vi "Callback Change Channel.vi"(8 "error in (no error)":errorcluster, 9 "old values":string[][](array[string]), 10 "object ref in":T1, 11 "Cluster":T2) -> (0 "error out":errorcluster, 6 "Variant":variant)   [LabVIEW 2013, in "Modbus Module editor node.lvclass"]
uses:
  Modbus Module editor node.lvclass
  <vilib>/NI/DCAF Table API/Table Manager/Cell Change.ctl
  <vilib>/NI/DCAF Table API/Table Manager/object ref.ctl
  <vilib>/NI/DCAF/Tag Editor Core/Configuration Editor/Classes/Engine Parent/Engine Parent Editor Node.lvclass
  <vilib>/NI/DCAF/Tag Editor Core/Configuration Editor/Classes/Module editor node/module editor node.lvclass
  module/configuration/Modbus Module configuration.lvclass
  <vilib>/NI/Configuration Framework/serializable configuration/NISE_CEF_serializable configuration.lvclass/NISE_CEF_serializable configuration.ctl
  <vilib>/NI/Tag Bus/tag/tag descriptor.lvclass/tag descriptor.ctl
  <vilib>/Utility/LVClass/Get LV Class Name.vi
  <vilib>/NI/Configuration Framework/error generator/NISE_error generator.vi
  <vilib>/NI/Module Execution Interface/Engine Configuration/engine configuration.lvclass
  <vilib>/NI/Configuration Framework/serializable configuration/NISE_CEF_serializable configuration.lvclass
  <vilib>/NI/Tag Bus/tag/tag descriptor.lvclass
  <vilib>/NI/DCAF Table API/Table Manager.lvlib
  <vilib>/NI/DCAF Table API/Table Manager/Table Manager.lvclass
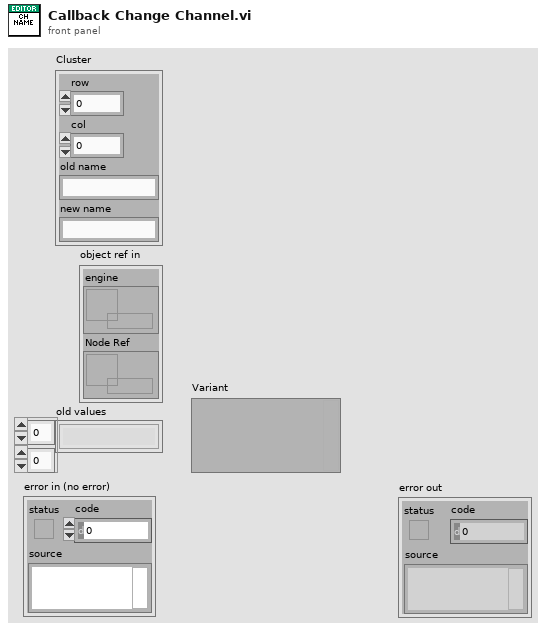
[diagram p1: front panel]
types:
  T1 = typedef "Table Manager.lvlib/Table Manager.lvclass/object ref.ctl" = cluster{"engine":refnum<data-value>, "Node Ref":refnum<data-value>}
  T2 = typedef "Table Manager.lvlib/Cell Change.ctl" = cluster{"row":i32, "col":i32, "old name":string, "new name":string}
  T3 = typedef "Modbus Module configuration.lvclass/Line.ctl" = refnum<class "Modbus Module Channel.lvclass">
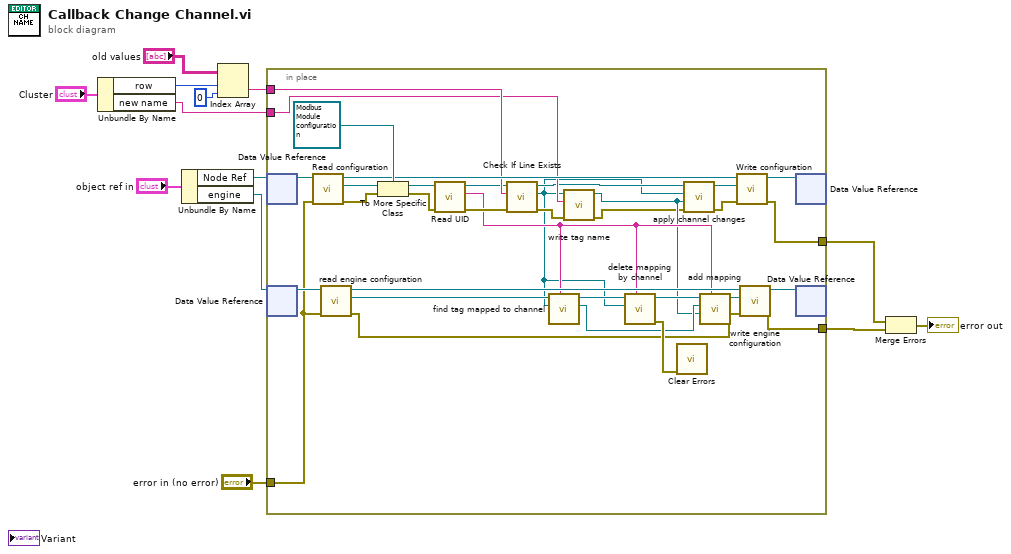
[diagram p0: block diagram]
diagram:
  n1 = Unbundle By Name("Cluster") -> ("row"=w7:i32, "new name"=w1:string)
  n2 = Unbundle By Name("object ref in") -> ("Node Ref"=w11:refnum<data-value>, "engine"=w10:refnum<data-value>)
  n3 = Index Array(array="old values", index (row)=w7, index (col)=0 ("disabled index (col)")) -> (element=w6:string)
  n4 = in-place {
    in-place-border: w6 -> [w38]
    in-place-border: "error in (no error)" -> [w28]
    in-place-border: [w30] -> w3
    in-place-border: [w29] -> w4
    in-place-border: w1 -> [w20]
    n5 = in-place-dvr #1(w11) -> (w43:refnum<class "module editor node.lvclass">)  [unwired: 1 out]
    n6 = in-place-dvr #2(w10) -> (w39:refnum<class "Engine Parent Editor Node.lvclass">)  [unwired: 1 out]
    n7 = call-dynamic "Read configuration.vi"("error in"=w28, "NISE_CEF_serializable node in"=w43) -> ("error out"=w31:errorcluster, "configuration"=w45:refnum<class "NISE_CEF_serializable configuration.lvclass">, "NISE_CEF_serializable node out"=w42:refnum<class "module editor node.lvclass">)  [unwired: 7 in]
    n8 = call <vilib>:"read engine configuration.vi"("error in"=w28, "Engine Parent Editor Node in"=w39) -> ("error out"=w27:errorcluster, "engine configuration"=w24:refnum<class "engine configuration.lvclass">, "Engine Parent Editor Node out"=w40:refnum<class "Engine Parent Editor Node.lvclass">)  [unwired: 7 in]
    n9 = To More Specific Class(target class=refnum<class "Modbus Module configuration.lvclass"> refnum ("Modbus Slave configuration in"), reference=w45, error in=w31) -> (specific class reference=w36:refnum<class "Modbus Module configuration.lvclass">, error out=w33:errorcluster)
    n10 = call <vilib>:"Read UID.vi"("error in"=w33, "configuration in"=w36) -> ("error out"=w32:errorcluster, "instance id"=w22:string, "configuration out"=w35:refnum<class "Modbus Module configuration.lvclass">)  [unwired: 7 in]
    n11 = call "Check If Line Exists.vi"("error in (no error)"=w32, "Name to locate"=w38, "Modbus Slave configuration in"=w35) -> ("error out"=w37:errorcluster, "Line out"=w14:T3, "Modbus Slave configuration out"=w19:refnum<class "Modbus Module configuration.lvclass">)  [unwired: 4 in, 2 out]
    n12 = call <vilib>:"find tag mapped to channel.vi"("owner"=w22, "channel"=w14, "engine configuration in"=w24) -> ("tag"=w21:refnum<class "tag descriptor.lvclass">, "engine configuration out"=w23:refnum<class "engine configuration.lvclass">)  [unwired: 6 in, 1 out]
    n13 = call <vilib>:"write tag name.vi"("error in"=w37, "name"=w20, "system tag in"=w14) -> ("error out"=w16:errorcluster, "system tag out"=w17:T3)  [unwired: 7 in]
    n14 = call <vilib>:"delete mapping by channel.vi"("owner ID"=w22, "channel"=w14, "engine configuration in"=w23) -> ("error out"=w34:errorcluster, "engine configuration out"=w26:refnum<class "engine configuration.lvclass">)  [unwired: 7 in]
    n15 = call <vilib>:"Clear Errors.vi"("error in (no error)"=w34) -> ()  [unwired: 6 in, 1 out]
    n16 = call "apply channel changes.vi"("error in"=w16, "new channel"=w17, "old channel"=w14, "Modbus Slave configuration in"=w19) -> ("error out"=w15:errorcluster, "Modbus Slave configuration out"=w18:refnum<class "Modbus Module configuration.lvclass">)  [unwired: 6 in]
    n17 = call <vilib>:"add mapping.vi"("owner ID"=w22, "channel"=w17, "tag descriptor"=w21, "engine configuration"=w26) -> ("engine configuration out"=w25:refnum<class "engine configuration.lvclass">)  [unwired: 6 in, 1 out]
    n18 = call-dynamic "Write configuration.vi"("error in"=w15, "configuration"=w18, "NISE_CEF_serializable node in"=w42) -> ("error out"=w29:errorcluster, "NISE_CEF_serializable node out"=w44:refnum<class "module editor node.lvclass">)  [unwired: 7 in]
    n19 = call <vilib>:"write engine configuration.vi"("error in"=w27, "engine configuration"=w25, "Engine Parent Editor Node in"=w40) -> ("error out"=w30:errorcluster, "Engine Parent Editor Node out"=w41:refnum<class "Engine Parent Editor Node.lvclass">)  [unwired: 7 in]
    n20 = in-place-dvr #1(w44) -> ()  [unwired: 2 out]
    n21 = in-place-dvr #2(w41) -> ()  [unwired: 2 out]
  }
  n22 = Merge Errors(w4, w3) -> (→"error out":errorcluster)
